vi "LogMessage.vi"(7 "eLogLvl":T1, 8 "Error":errorcluster[](array[cluster]), 11 "LogMessage":string) -> (0 "Error":errorcluster[](array[cluster]))   [LabVIEW 2018]
uses:
  LV_Config_class/Typedefs/eLogLvl.ctl
  LV_Config_class/Config.lvclass/Config.ctl
  LV_Config_class/Accessors/Read Logging.vi
  LV_Config_class/Config.lvclass
  <userlib>/NIST/NISTErrorLib/NISTErrorLib.lvlib
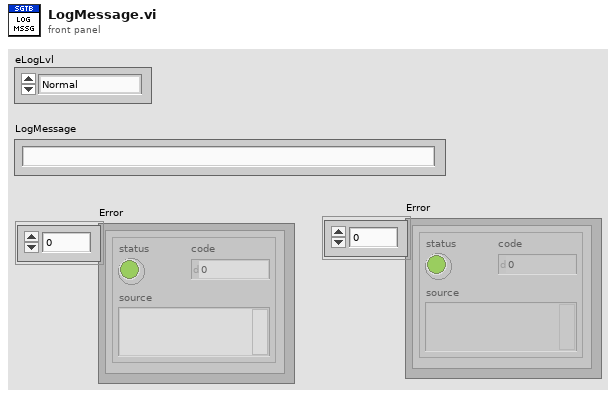
[diagram p1: front panel]
types:
  T1 = typedef "Config_class.lvlib/Config.lvclass/eLogLvl.ctl" = enum16{"Normal", "Verbose", "None"}
  T2 = typedef "Config_class.lvlib/Config.lvclass/Logging.ctl" = cluster{"eLogLvl":T1, "Log File Path":path, "btnLogFile":bool}
  T3 = enum16{"open", "replace", "create", "open or create", "replace or create", "replace or create with confirmation"}
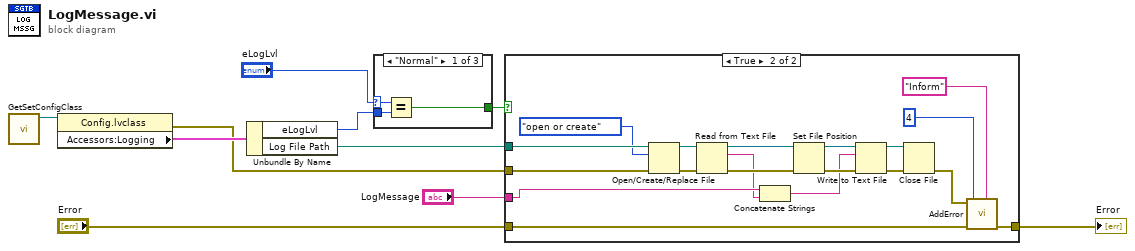
[diagram p0: block diagram]
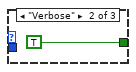
[diagram p2: hidden frame]
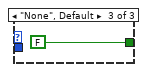
[diagram p3: hidden frame]
diagram:
  n1 = call "GetSetConfigClass.vi"() -> ("Ref out"=w10:refnum<class "Config.lvclass">)  [unwired: 11 in]
  n2 = property class="Config.lvclass"(reference=w10) -> (error out=w6:errorcluster, "Accessors:Logging"=w9:T2)  [unwired: 1 in, 1 out]
  n3 = Unbundle By Name(w9) -> ("eLogLvl"=w2:T1, "Log File Path"=w5:path)
  n4 = case shown="\"Normal\"" "eLogLvl" {
    selector: "eLogLvl" -> [w12 _ _]
    tunnel: [w13 TRUE FALSE] -> w3
    tunnel: w2 -> [w11 _ _]
    frame "Normal" {
      n5 = Equal?(x=w12, y=w11) -> (x = y?=w13:bool)
    }
    frame "Verbose" {
    }
    frame "None", Default {
    }
  }
  n6 = case shown="True" w3 {
    tunnel: w5 -> [_ w35]
    tunnel: [w16 w34] -> w7
    tunnel: "Error" -> [w16 w28]
    tunnel: "LogMessage" -> [_ w18]
    tunnel: w6 -> [_ w23]
    frame False {
    }
    frame True {
      n7 = Open/Create/Replace File(file path (use dialog)=w35, error in=w23, operation (0:open)=T3."open or create") -> (refnum out=w21:refnum<file>, error out=w24:errorcluster)  [unwired: 3 in, 1 out]
      n8 = Read from Text File(file (use dialog)=w21, error in=w24) -> (refnum out=w20:refnum<file>, text=w17:string, error out=w22:errorcluster)  [unwired: 2 in, 1 out]
      n9 = Concatenate Strings(w18, w17) -> (w19:string)
      n10 = Set File Position(refnum=w20, error in=w22) -> (refnum out=w27:refnum<file>, error out=w26:errorcluster)  [unwired: 2 in]
      n11 = Write to Text File(file (use dialog)=w27, text=w19, error in=w26) -> (refnum out=w32:refnum<file>, error out=w33:errorcluster)  [unwired: 1 in, 1 out]
      n12 = Close File(refnum=w32, error in=w33) -> (error out=w31:errorcluster)  [unwired: 1 out]
      n13 = call <userlib>:"AddError.vi"("Severity"="Inform", "Priority"=u8 4, "ErrorArray"=w28, "error in (no error)"=w31) -> ("ErrorArray"=w34:errorcluster[])  [unwired: 6 in, 1 out]
    }
  }
  "Error" <- w7
